vi "SRV_FOR_Start.vi"(0 "N":string="5", 2 "SuperPro":T1) -> (1 "Counter":string, 4 "SuperPro":T1)   [LabVIEW 2009]
doc: "Starts a loop that runs N times. N can be specified as a number or a variable (string). You can also define the loop counter (default is i)."
uses:
  <userlib>/SuperPro/OpCodes/_SubVIs/SuperProControl.ctl
panel:
  # "This LabVIEW item is deprecated.\n\nIt is believed to be unused and will be removed in a future version of SRV."
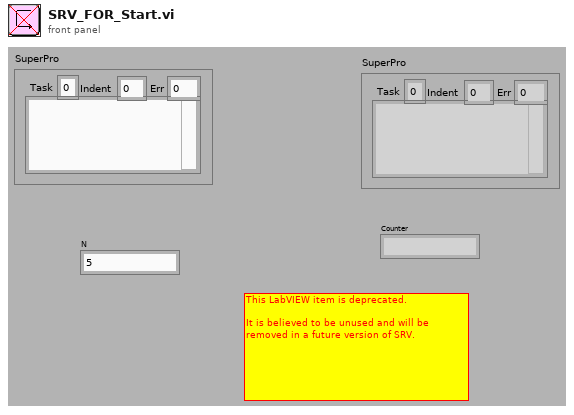
[diagram p1: front panel]
types:
  T1 = typedef "SuperProControl.ctl" = cluster{"Task":i32, "Indent":i32, "Err":i32, "ASM":string}
  T2 = enum16{"boolean", "u8", "i8", "u16", "i16", "u32", "i32", "u64", "i64", "SGL", "DBL", "EXT", "CPX"}
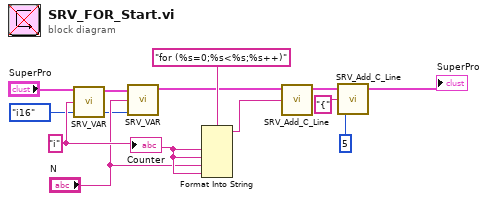
[diagram p0: block diagram]
diagram:
  w1 = T2."i16" ("type")
  w3 = "i" ("Counter")
  n1 = call "SRV_VAR.vi"("SuperPro in"="SuperPro", "Name"=w3, "type"=w1) -> ("SuperPro out"=w5:T1)  [unwired: 3 out]
  n2 = call "SRV_VAR.vi"("SuperPro in"=w5, "Name"="N", "type"=w1) -> ("SuperPro out"=w4:T1)  [unwired: 3 out]
  n3 = Format Into String(format string="for (%s=0;%s<%s;%s++)", w3, w3, "N", w3) -> (resulting string=w11:string)  [unwired: 2 in, 1 out]
  n4 = call "SRV_Add_C_Line.vi"("C String"=w11, "SuperPro in"=w4) -> ("SuperPro out"=w10:T1)  [unwired: 3 in]
  n5 = call "SRV_Add_C_Line.vi"("inc"=5 ("y"), "C String"="{" ("format string"), "SuperPro in"=w10) -> ("SuperPro out"=→"SuperPro":T1)  [unwired: 2 in]
  "Counter" <- w3
